vi "get_dev_names.vi"(8 "error in (no error)":errorcluster) -> (0 "error out":errorcluster, 3 "DevNames":tag[](array[tag]))   [LabVIEW 2015]
uses:
  <resource>/objmgr/daqmx.rc
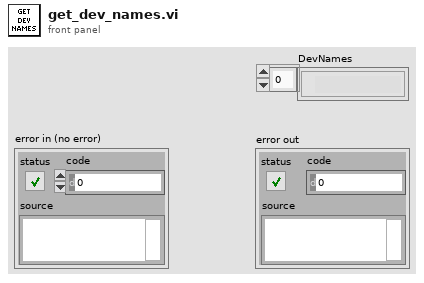
[diagram p1: front panel]
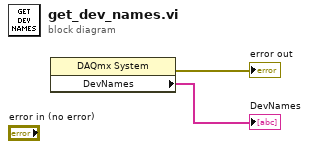
[diagram p0: block diagram]
diagram:
  n1 = property class="DAQmx System"() -> (error out=→"error out":errorcluster, "DevNames"=→"DevNames":tag[])  [unwired: 2 in, 1 out]
